vi "Periodic Tasks.vi"(7 "Chassis X SPD":dbl=0.65, 8 "error in":errorcluster) -> ()   [LabVIEW 2019]
doc: "This VI runs in parallel to other tasks. It can contain as many user-defined periodic loops as you need. These can carry out PID or other sorts of timed response."
uses:
  Robot Global Data.vi
  <vilib>/Rock Robotics/Network Tables/NT Write Number.vi
  <vilib>/Rock Robotics/Network Tables/NT Read Number.vi
  <vilib>/Rock Robotics/WPI/RobotDrive/WPI_RobotDriveArcadeDrive_Standard(NoSaturation).vi
  <vilib>/Rock Robotics/Network Tables/NT Read Boolean.vi
panel:
  in  "h1":dbl
  in  "a1":dbl
  in  "Chassis Y SPD":dbl=0.65
  # "The tilt applied to the Limelight when mounted"
  # "Height of the floor to the center of the limelight"
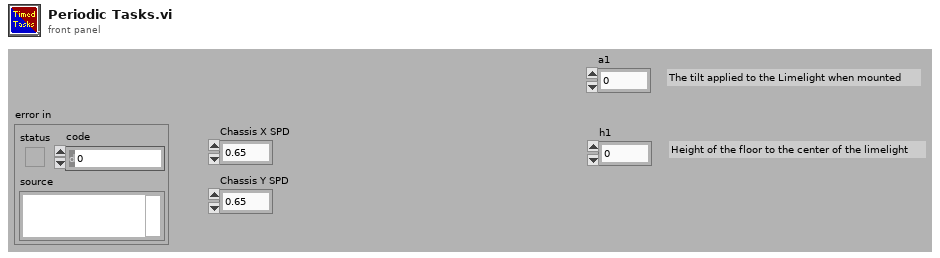
[diagram p1: front panel]
types:
  T1 = typedef "WPI_JoystickDevRef.ctl" = cluster{"Device":T2}
  T2 = typedef "WPI_JoystickDeviceEnum.ctl" = enum16{"USB 0", "USB 1", "USB 2", "USB 3", "USB 4", "USB 5"}
  T3 = typedef "WPI_RobotDriveDevRef.ctl" = cluster{"DevStatus":errorcluster, "Motors[]":T4[], "Square Inputs":bool, "Max Output":dbl}
  T4 = typedef "WPI_MotorControlDeviceRef.ctl" = cluster{"DeviceStatus":errorcluster, "Type":T5, "PWM":cluster{"PWM Channel":T6, "DeadBand":T7}, "CAN":cluster{"Device Number":u8, "SetOutput VI Ref":variant, "GetOutput VI Ref":variant, "Enable VI Ref":variant, "Disable VI Ref":variant, "Data":variant}, "Invert":bool, "DIO PWM":cluster{"PWM \"Enable\" Channel":T6, "DIOChannel":T8, "PWM Rate":dbl}}
  T5 = typedef "WPI_MotorControlType.ctl" = enum16{"PWM", "CAN", "DIO PWM"}
  T6 = typedef "FPGA_DIOPWMChannel.ctl" = enum8{"PWM 0", "PWM 1", "PWM 2", "PWM 3", "PWM 4", "PWM 5", "PWM 6", "PWM 7", "PWM 8", "PWM 9", "PWM MXP 0", "PWM MXP 1", "PWM MXP 2", "PWM MXP 3", "PWM MXP 4", "PWM MXP 5", "PWM MXP 6", "PWM MXP 7", "PWM MXP 8", "PWM MXP 9", "Invalid"}
  T7 = typedef "WPI_PWMDeadband.ctl" = cluster{"Name":string, "maxPositivePwm":i32, "minPositivePwm":i32, "centerPwm":i32, "maxNegativePwm":i32, "minNegativePwm":i32, "angularRange":u16}
  T8 = typedef "FPGA_DIOChannel.ctl" = enum8{"DIO 0", "DIO 1", "DIO 2", "DIO 3", "DIO 4", "DIO 5", "DIO 6", "DIO 7", "DIO 8", "DIO 9", "DIO MXP 0", "DIO MXP 1", "DIO MXP 2", "DIO MXP 3", "DIO MXP 4", "DIO MXP 5", "DIO MXP 6", "DIO MXP 7", "DIO MXP 8", "DIO MXP 9", "DIO MXP 10", "DIO MXP 11", "DIO MXP 12", "DIO MXP 13", "DIO MXP 14", "DIO MXP 15", "SPI Port CS1", "SPI Port CS2", "SPI Port CS3", "SPI Port MISO", "SPI Port MOSI", "Invalid"}
  T9 = cluster{"JoystickDevRef":T1, "RobotDriveDevRef":T3}
  T10 = typedef "WPI_ServoDeviceRef.ctl" = cluster{"DeviceStatus":errorcluster, "PWM Channel":T6, "DeadBand":T7}
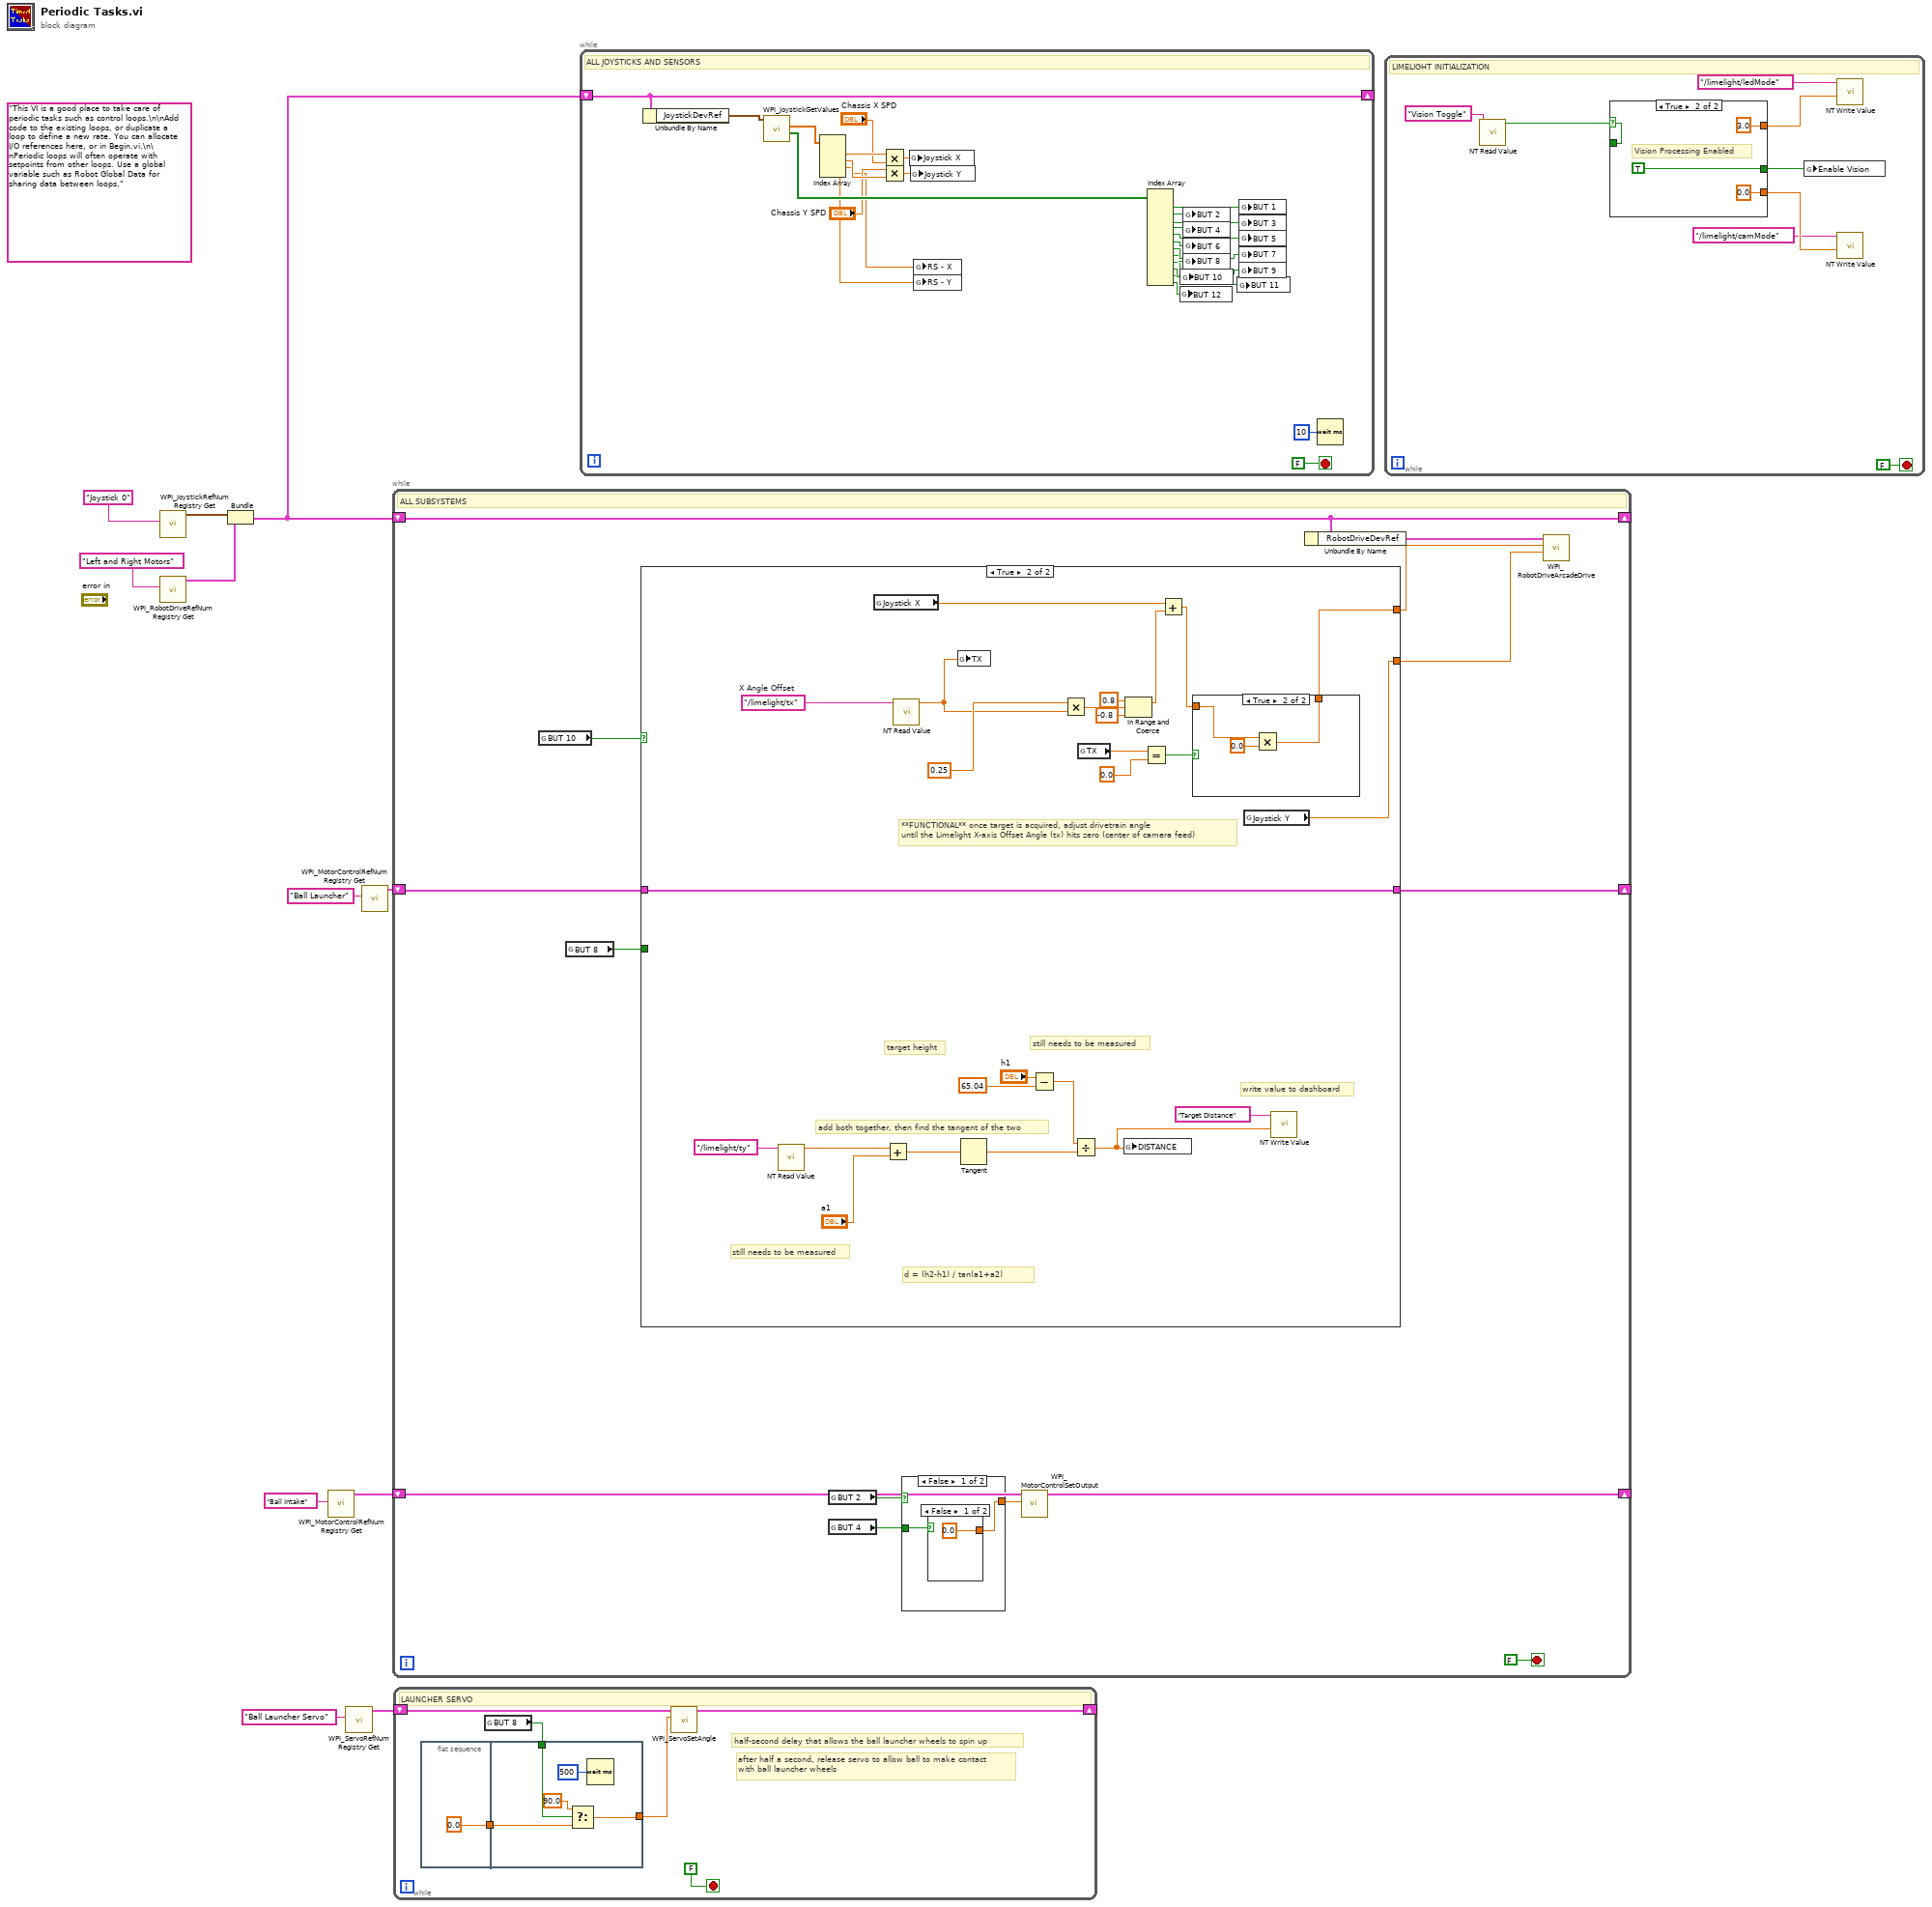
[diagram p0: block diagram]
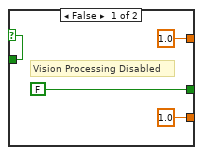
[diagram p2: hidden frame]
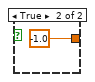
[diagram p3: hidden frame]
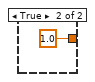
[diagram p4: hidden frame]
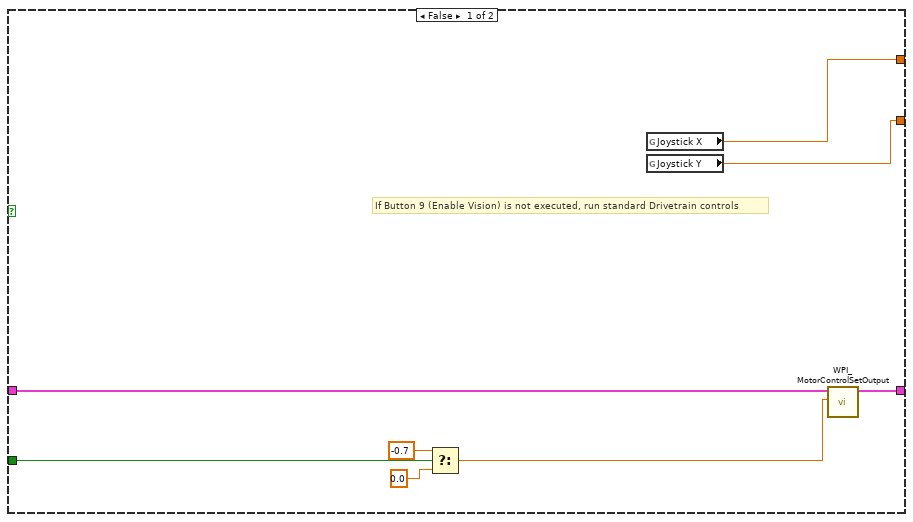
[diagram p5: hidden frame]
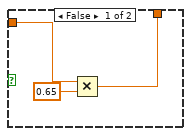
[diagram p6: hidden frame]
diagram:
  (unwired) "This VI is a good place to take care of periodic tasks such as control loops.\n\nAdd code to the existing loops, or duplicate a loop to define a new rate. You can allocate I/O references here, or in Begin.vi.\n\nPeriodic loops will often operate with setpoints from other loops. Use a global variable such as Robot Global Data for sharing data between loops."
  n1 = call <vilib>:"WPI_JoystickRefNum Registry Get.vi"("refnum name"="Joystick 0") -> ("JoystickDevRef"=w9:T1)  [unwired: 1 in, 9 out]
  n2 = call <vilib>:"WPI_RobotDriveRefNum Registry Get.vi"("refnum name"="Left and Right Motors") -> ("RobotDriveDevRef"=w8:T3)  [unwired: 1 in, 9 out]
  n3 = Bundle("JoystickDevRef"=w9, "RobotDriveDevRef"=w8) -> (w7:T9)  [unwired: 1 out]
  n4 = call <vilib>:"WPI_MotorControlRefNum Registry Get.vi"("refnum name"="Ball Intake") -> ("MotorControlDevRef"=w2:T4)  [unwired: 9 in, 1 out]
  n5 = call <vilib>:"WPI_ServoRefNum Registry Get.vi"("refnum name"="Ball Launcher Servo") -> ("ServoDeviceRef"=w4:T10)  [unwired: 9 in, 1 out]
  n6 = call <vilib>:"WPI_MotorControlRefNum Registry Get.vi"("refnum name"="Ball Launcher") -> ("MotorControlDevRef"=w6:T4)  [unwired: 9 in, 1 out]
  n7 = while {
    shift-right: [w24] -> _
    shift-left: w7 -> [w24]
    shift-right: [w17] -> _
    shift-left: w6 -> [w18]
    shift-right: [w13] -> _
    shift-left: w2 -> [w12]
    stop <- FALSE stop-if-true
    # "ALL SUBSYSTEMS"
    n8 = global read "Robot Global Data.vi" "BUT 10"() -> (w23:bool)
    n9 = global read "Robot Global Data.vi" "BUT 8"() -> (w19:bool)
    n10 = case shown="True" w23 {
      tunnel: [w38 w54] -> w21
      tunnel: [w37 w50] -> w20
      tunnel: w19 -> [w32 _]
      tunnel: w18 -> [w35 w39]
      tunnel: [w36 w39] -> w17
      frame False {
        # "If Button 9 (Enable Vision) is not executed, run standard Drivetrain controls"
        n11 = Select(t=-0.7, s=w32, f=0.0) -> (s? t:f=w34:dbl)
        n12 = global read "Robot Global Data.vi" "Joystick X"() -> (w38:dbl)
        n13 = global read "Robot Global Data.vi" "Joystick Y"() -> (w37:dbl)
        n14 = call <vilib>:"WPI_MotorControlSetOutput.vi"("Output"=w34, "MotorControlDevRef"=w35) -> ("MotorControlDevRef"=w36:T4)  [unwired: 7 in, 2 out]
      }
      frame True {
        w63 = "/limelight/tx"  # X Angle Offset
        # "write value to dashboard"
        # "still needs to be measured"
        # "target height"
        # "add both together, then find the tangent of the two"
        # "still needs to be measured"
        # "d = (h2-h1) / tan(a1+a2)"
        # "**FUNCTIONAL** once target is acquired, adjust drivetrain angle \nuntil the Limelight X-axis Offset Angle (tx) hits zero (center of camera feed)"
        n15 = call-poly <vilib>:"NT Read Value.vi"("Name"="/limelight/ty") -> ("Numeric"=w48:dbl)  [unwired: 9 in, 1 out]
        n16 = global read "Robot Global Data.vi" "Joystick X"() -> (w62:dbl)
        n17 = Add(x=w48, y="a1") -> (x+y=w46:dbl)
        n18 = call-poly <vilib>:"NT Read Value.vi"("Name"=w63) -> ("Numeric"=w56:dbl)  [unwired: 9 in, 1 out]
        n19 = global write "Robot Global Data.vi" "TX"(w56) -> ()
        n20 = Tangent(1:w46) -> (0:w45:dbl)
        n21 = Subtract(x="h1", y=65.04) -> (x-y=w43:dbl)
        n22 = Multiply(x=0.25 ("y"), y=w56) -> (x*y=w60:dbl)
        n23 = Divide(x=w43, y=w45) -> (x/y=w40:dbl)
        n24 = global read "Robot Global Data.vi" "TX"() -> (w52:dbl)
        n25 = global write "Robot Global Data.vi" "DISTANCE"(w40) -> ()
        n26 = In Range and Coerce(upper limit=0.8, x=w60, lower limit=-0.8) -> (coerced(x)=w61:dbl)  [unwired: 1 out]
        n27 = Equal?(x=w52, y=0.0) -> (x = y?=w53:bool)
        n28 = Add(x=w62, y=w61) -> (x+y=w55:dbl)
        n29 = case shown="True" w53 {
          tunnel: w55 -> [w65 w69]
          tunnel: [w66 w67] -> w54
          frame False {
            n30 = Multiply(x=w65, y=0.65) -> (x*y=w66:dbl)
          }
          frame True {
            n31 = Multiply(x=w69, y=0.0) -> (x*y=w67:dbl)
          }
        }
        n32 = global read "Robot Global Data.vi" "Joystick Y"() -> (w50:dbl)
        n33 = call-poly <vilib>:"NT Write Value.vi"("Numeric"=w40, "Name"="Target Distance") -> ()  [unwired: 9 in, 1 out]
      }
    }
    n34 = global read "Robot Global Data.vi" "BUT 2"() -> (w15:bool)
    n35 = global read "Robot Global Data.vi" "BUT 4"() -> (w16:bool)
    n36 = case shown="False" w15 {
      tunnel: [w27 1.0 ("Output")] -> w14
      tunnel: w16 -> [w26 _]
      frame False {
        n37 = case shown="False" w26 {
          tunnel: [0.0 ("Output") -1.0 ("Output")] -> w27
          frame False {
          }
          frame True {
          }
        }
      }
      frame True {
      }
    }
    n38 = call <vilib>:"WPI_MotorControlSetOutput.vi"("Output"=w14, "MotorControlDevRef"=w12) -> ("MotorControlDevRef"=w13:T4)  [unwired: 7 in, 2 out]
    n39 = Unbundle By Name(w24) -> ("RobotDriveDevRef"=w22:T3)
    n40 = call-poly <vilib>:"WPI_RobotDriveArcadeDrive.vi"("Y axis value"=w20, "X axis value"=w21, "RobotDriveDevRef"=w22) -> ()  [unwired: 6 in, 3 out]
  }
  n41 = while {
    shift-right: [w71] -> _
    shift-left: w4 -> [w72]
    stop <- FALSE stop-if-true
    # "after half a second, release servo to allow ball to make contact\nwith ball launcher wheels"
    # "half-second delay that allows the ball launcher wheels to spin up"
    # "LAUNCHER SERVO"
    n42 = flat-sequence {
      tunnel: [0.0 ("f")] -> w75
      tunnel: [w80] -> w74
      tunnel: w73 -> [w79]
      tunnel: w75 -> [w77]
      frame #0 {
      }
      frame #1 {
        n43 = Select(t=90.0, s=w79, f=w77) -> (s? t:f=w80:dbl)
        n44 = Wait (ms)(milliseconds to wait=u32 500) -> ()  [unwired: 1 out]
      }
    }
    n45 = global read "Robot Global Data.vi" "BUT 8"() -> (w73:bool)
    n46 = call <vilib>:"WPI_ServoSetAngle.vi"("Angle"=w74, "ServoDeviceRef"=w72) -> ("ServoDeviceRef"=w71:T10)  [unwired: 8 in, 1 out]
  }
  n47 = while {
    shift-right: [w91] -> _
    shift-left: w7 -> [w91]
    stop <- FALSE stop-if-true
    # "ALL JOYSTICKS AND SENSORS"
    n48 = Unbundle By Name(w91) -> ("JoystickDevRef"=w105:T1)
    n49 = call <vilib>:"WPI_JoystickGetValues.vi"("JoystickDevRef"=w105) -> ("Buttons"=w104:bool[], "Axes"=w90:dbl[])  [unwired: 6 in, 3 out]
    n50 = Index Array(array=w90) -> (element #1=w87:dbl, element #2=w86:dbl, element #3=w83:dbl, element #4=w82:dbl)  [unwired: 4 in]
    n51 = Multiply(x=w87, y="Chassis X SPD") -> (x*y=w89:dbl)
    n52 = Multiply(x="Chassis Y SPD", y=w86) -> (x*y=w88:dbl)
    n53 = global write "Robot Global Data.vi" "Joystick X"(w89) -> ()
    n54 = global write "Robot Global Data.vi" "Joystick Y"(w88) -> ()
    n55 = global write "Robot Global Data.vi" "RS - X"(w83) -> ()
    n56 = global write "Robot Global Data.vi" "RS - Y"(w82) -> ()
    n57 = Index Array(array=w104) -> (element #1=w103:bool, element #2=w102:bool, element #3=w101:bool, element #4=w100:bool, element #5=w99:bool, element #6=w98:bool, element #7=w97:bool, element #8=w96:bool, element #9=w95:bool, element #10=w94:bool, element #11=w93:bool, element #12=w92:bool)  [unwired: 12 in]
    n58 = global write "Robot Global Data.vi" "BUT 12"(w92) -> ()
    n59 = global write "Robot Global Data.vi" "BUT 10"(w94) -> ()
    n60 = global write "Robot Global Data.vi" "BUT 2"(w102) -> ()
    n61 = global write "Robot Global Data.vi" "BUT 4"(w100) -> ()
    n62 = global write "Robot Global Data.vi" "BUT 6"(w98) -> ()
    n63 = global write "Robot Global Data.vi" "BUT 8"(w96) -> ()
    n64 = global write "Robot Global Data.vi" "BUT 11"(w93) -> ()
    n65 = global write "Robot Global Data.vi" "BUT 1"(w103) -> ()
    n66 = global write "Robot Global Data.vi" "BUT 3"(w101) -> ()
    n67 = global write "Robot Global Data.vi" "BUT 5"(w99) -> ()
    n68 = global write "Robot Global Data.vi" "BUT 7"(w97) -> ()
    n69 = global write "Robot Global Data.vi" "BUT 9"(w95) -> ()
    n70 = Wait (ms)(milliseconds to wait=u32 10) -> ()  [unwired: 1 out]
  }
  n71 = while {
    stop <- FALSE stop-if-true
    # "LIMELIGHT INITIALIZATION"
    n72 = call-poly <vilib>:"NT Read Value.vi"("Name"="Vision Toggle") -> ("Boolean"=w109:bool)  [unwired: 9 in, 1 out]
    n73 = case shown="True" w109 {
      selector: w109 -> [w116 w120]
      tunnel: [FALSE ("Enable Vision") TRUE ("Enable Vision")] -> w113
      tunnel: [1.0 ("Numeric") 0.0 ("Numeric")] -> w114
      tunnel: [1.0 ("Numeric") 3.0 ("Numeric")] -> w115
      tunnel: [w116 w120] -> _
      frame False {
        # "Vision Processing Disabled"
      }
      frame True {
        # "Vision Processing Enabled"
      }
    }
    n74 = global write "Robot Global Data.vi" "Enable Vision"(w113) -> ()
    n75 = call-poly <vilib>:"NT Write Value.vi"("Numeric"=w115, "Name"="/limelight/ledMode") -> ()  [unwired: 9 in, 1 out]
    n76 = call-poly <vilib>:"NT Write Value.vi"("Numeric"=w114, "Name"="/limelight/camMode") -> ()  [unwired: 9 in, 1 out]
  }
